vi "Speed&Length_Calculator.vi"(0 "Sensors_Distance [mm]":u32=101, 1 "TriggerS1":bool, 2 "TriggerS2":bool, 3 "Max_Time [ms]":u32) -> (4 "Flag_EndMeasure":bool, 5 "Speed [m/s]":dbl, 6 "Length [mm]":dbl, 7 "Alarm":bool)   [LabVIEW 2020]
panel:
  out "Stop_T2 [ms]":u32
  out "Start_T2 [ms]":u32
  out "Stop_T1 [ms]":u32
  out "Start_T1 [ms]":u32
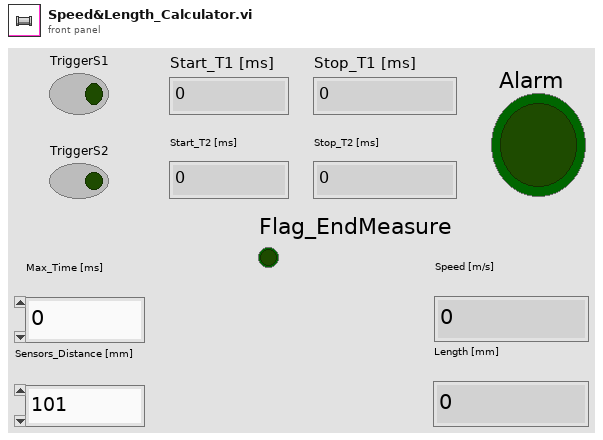
[diagram p1: front panel]
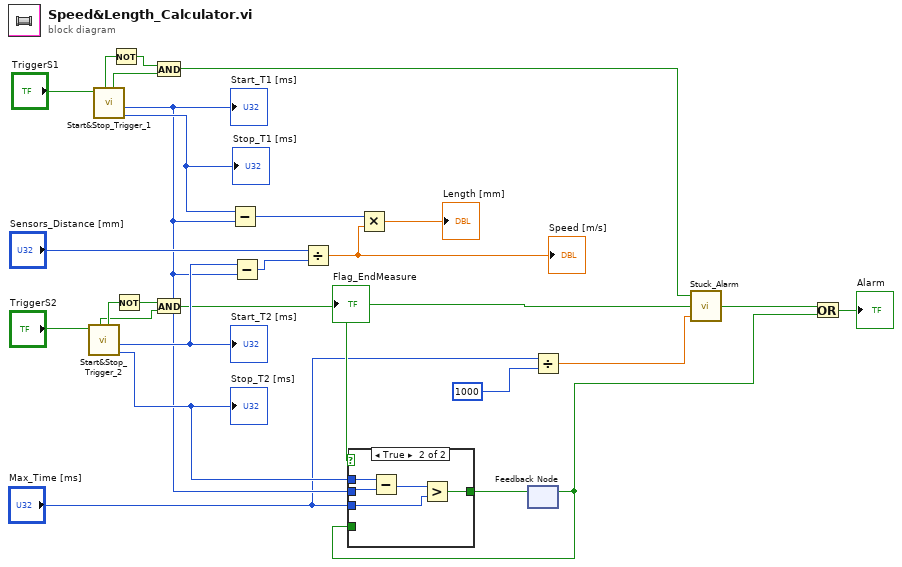
[diagram p0: block diagram]
diagram:
  n1 = call "Start&Stop_Trigger_2.vi"("TriggerSn"="TriggerS2") -> ("Stop_Tn"=w14:u32, "Start_Tn"=w22:u32, "TriggerSn_prev0"=w16:bool, "TriggerSn_prev-1"=w15:bool)  [unwired: 5 in, 2 out]
  "Start_T2 [ms]" <- w22
  "Stop_T2 [ms]" <- w14
  n2 = call "Start&Stop_Trigger_1.vi"("TriggerSn"="TriggerS1") -> ("Stop_Tn"=w24:u32, "Start_Tn"=w13:u32, "TriggerSn_prev0"=w1:bool, "TriggerSn_prev-1"=w3:bool)  [unwired: 5 in, 2 out]
  "Start_T1 [ms]" <- w13
  "Stop_T1 [ms]" <- w24
  n3 = Not(x=w3) -> (.not. x?=w2:bool)
  n4 = Not(x=w16) -> (.not. x?=w17:bool)
  n5 = And(x=w2, y=w1) -> (x .and. y?=w11:bool)
  n6 = And(x=w17, y=w15) -> (x .and. y?=w10:bool)
  "Flag_EndMeasure" <- w10
  n7 = Subtract(x=w24, y=w13) -> (x-y=w23:u32)
  n8 = Subtract(x=w22, y=w13) -> (x-y=w20:u32)
  n9 = Divide(x="Sensors_Distance [mm]", y=w20) -> (x/y=w19:dbl)
  "Speed [m/s]" <- w19
  n10 = Multiply(x=w23, y=w19) -> (x*y=→"Length [mm]":dbl)
  n11 = feedback #1() -> (w5:bool)  [unwired: 1 in]
  n12 = case shown="True" w10 {
    tunnel: w14 -> [_ w32]
    tunnel: w13 -> [_ w31]
    tunnel: "Max_Time [ms]" -> [_ w29]
    tunnel: [w27 w28] -> w12
    tunnel: w5 -> [w27 _]
    frame False {
    }
    frame True {
      n13 = Subtract(x=w32, y=w31) -> (x-y=w30:u32)
      n14 = Greater?(x=w30, y=w29) -> (0:w28:bool)
    }
  }
  n15 = feedback-in #1(w12) -> ()
  n16 = Divide(x="Max_Time [ms]", y=u32 1000) -> (x/y=w7:dbl)
  n17 = call "Stuck_Alarm.vi"("Time Target (s)"=w7, "Finish_Measurement"=w10, "Start_Measurement"=w11) -> ("Stuck_Alarm"=w6:bool)
  n18 = Or(x=w6, y=w5) -> (x .or. y?=→"Alarm":bool)
